vi "Rotate_Coordinate.vi"(2 "Input Data":dbl[](array[numeric]), 3 "Rotation Angle":dbl) -> (0 "Rotated Data":dbl[](array[numeric]) format="%.2f", 1 "Rotation Matrix":T1)   [LabVIEW 2011]
uses:
  <vilib>/Analysis/Matrix/Datatypes/RealMatrix.ctl
  <vilib>/Analysis/baseanly.llb/A x Vector.vi
  <vilib>/Analysis/NI_AALBase.lvlib
  <vilib>/Analysis/Matrix/NI_Matrix.lvlib
panel:
  # "X"
  # "="
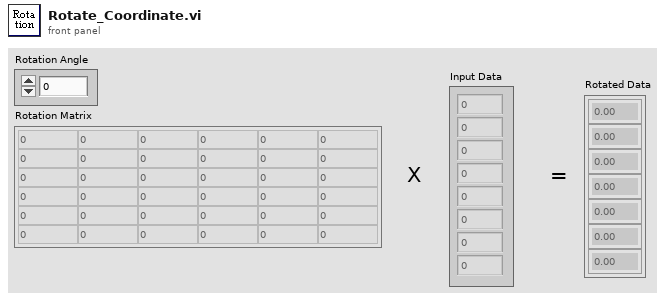
[diagram p1: front panel]
types:
  T1 = typedef "NI_Matrix.lvlib/RealMatrix.ctl" = dbl[][]
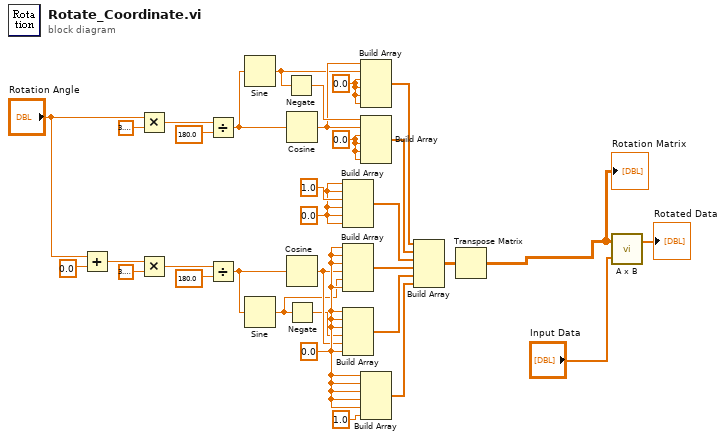
[diagram p0: block diagram]
diagram:
  w22 = 0.0 ("원소")
  w28 = 0.0 ("원소")
  w18 = 0.0 ("원소")
  w17 = 0.0 ("원소")
  n1 = Add(x="Rotation Angle", y=0.0 ("x")) -> (x+y=w5:dbl)
  n2 = Multiply(x="Rotation Angle", y=3.141592653589793) -> (x*y=w33:dbl)
  n3 = Multiply(x=w5, y=3.141592653589793) -> (x*y=w8:dbl)
  n4 = Divide(x=w33, y=180.0 ("x")) -> (x/y=w30:dbl)
  n5 = Divide(x=w8, y=180.0 ("x")) -> (x/y=w11:dbl)
  n6 = Sine(x=w30) -> (sin(x)=w12:dbl)
  n7 = Sine(x=w11) -> (sin(x)=w2:dbl)
  n8 = Negate(x=w12) -> (-x=w14:dbl)
  n9 = Cosine(x=w30) -> (cos(x)=w13:dbl)
  n10 = Cosine(x=w11) -> (cos(x)=w4:dbl)
  n11 = Negate(x=w2) -> (-x=w3:dbl)
  n12 = Build Array(w28, w28, 1.0 ("원소"), w28, w28, w28) -> (w25:dbl[])
  n13 = Build Array(w22, w22, w22, w4, w2, w22) -> (w21:dbl[])
  n14 = Build Array(w22, w22, w22, w3, w4, w22) -> (w20:dbl[])
  n15 = Build Array(w13, w12, w17, w17, w17, w17) -> (w27:dbl[])
  n16 = Build Array(w14, w13, w18, w18, w18, w18) -> (w26:dbl[])
  n17 = Build Array(w22, w22, w22, w22, w22, 1.0 ("원소")) -> (w19:dbl[])
  n18 = Build Array(w27, w26, w25, w21, w20, w19) -> (w24:T1)
  n19 = Transpose Matrix(1:w24) -> (0:w1:T1)
  "Rotation Matrix" <- w1
  n20 = call-poly <vilib>:"A x B.vi"("Vector"="Input Data", "A"=w1) -> ("A x Vector"=→"Rotated Data":dbl[])  [unwired: 1 out]
